vi "Get Exposure Time.vi"(8 "error in (no error)":errorcluster) -> (0 "error out":errorcluster, 2 "Exposure (ms)":u16)   [LabVIEW 2017]
doc: "Returns the exposure time in ms."
uses:
  HighFinesse WS5/wlmData.dll
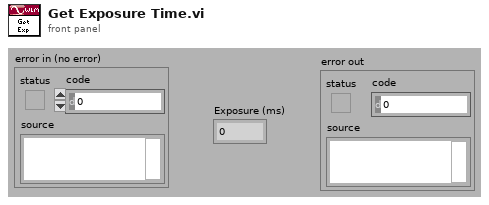
[diagram p1: front panel]
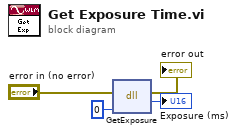
[diagram p0: block diagram]
diagram:
  n1 = dll-call lib="C:/LabVIEW-programs-dev/Instruments/Wavelength meter/HighFinesse WS5/wlmData.dll" fn="GetExposure"(error in="error in (no error)", "E"=u16 0) -> (error out=→"error out":errorcluster, "return type"=→"Exposure (ms)":u16)  [unwired: 3 in, 1 out]
